vi "GetTrendNames.vi"(11 "AssetNodes":T1[](array[typedef])) -> (3 "trend names":variant)   [LabVIEW 2016]
doc: "Processes the asset nodes for the trend names."
uses:
  <vilib>/addons/InsightCM/Utilities/DeviceModelHelpers/DeviceModelHelpers.lvlib
  <vilib>/addons/InsightCM/MessageBus/Base/controls/AssetState.ctl
  <vilib>/addons/InsightCM/MessageBus/Base/controls/KeyValuePair.ctl
  <vilib>/addons/InsightCM/MessageBus/Base/controls/Metric.ctl
  <vilib>/addons/InsightCM/MessageBus/Base/controls/AssetNodeReference.ctl
  <vilib>/addons/InsightCM/MessageBus/Base/controls/AssetNodeView.ctl
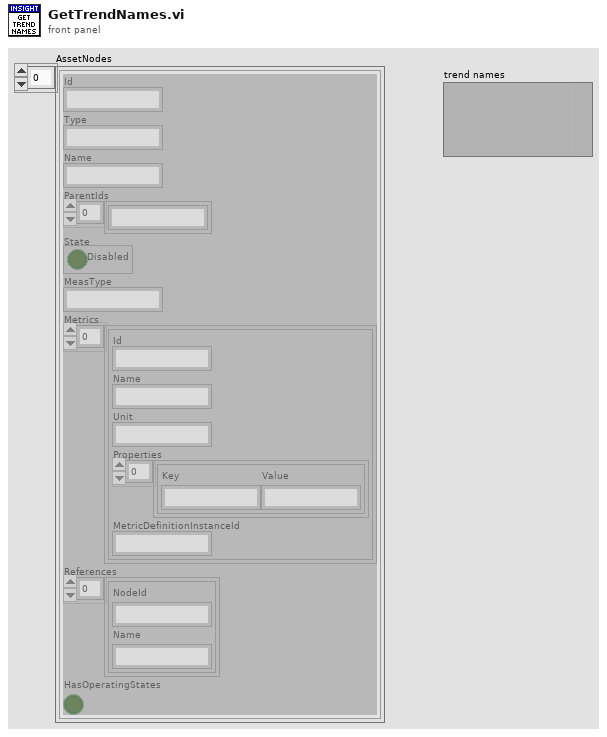
[diagram p1: front panel]
types:
  T1 = typedef "AssetNodeView.ctl" = cluster{"Id":string, "Type":string, "Name":string, "ParentIds":string[], "State":T2, "MeasType":string, "Metrics":T3[], "References":T5[], "HasOperatingStates":bool}
  T2 = typedef "AssetState.ctl" = cluster{"Disabled":bool}
  T3 = typedef "Metric.ctl" = cluster{"Id":string, "Name":string, "Unit":string, "Properties":T4[], "MetricDefinitionInstanceId":string}
  T4 = typedef "KeyValuePair.ctl" = cluster{"Key":string, "Value":string}
  T5 = typedef "AssetNodeReference.ctl" = cluster{"NodeId":string, "Name":string}
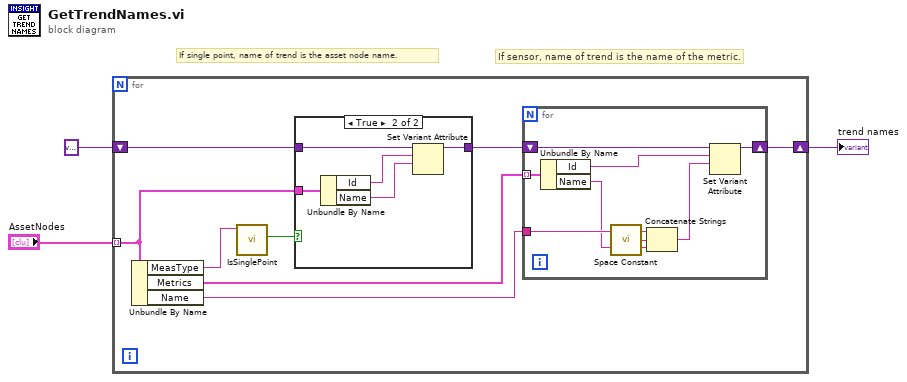
[diagram p0: block diagram]
diagram:
  # "If sensor, name of trend is the name of the metric."
  # "If single point, name of trend is the asset node name."
  n1 = for {
    tunnel: "AssetNodes" -> [w8] mode=indexing
    shift-right: [w6] -> w1
    shift-left: variant ("trend names") -> [w9]
    n2 = Unbundle By Name(w8) -> ("MeasType"=w11:string, "Metrics"=w5:T3[], "Name"=w4:string)
    n3 = call <vilib>:"IsSinglePoint.vi"("MeasType"=w11) -> ("is single point"=w10:bool)  [unwired: 10 in]
    n4 = case shown="True" w10 {
      tunnel: w9 -> [w12 w17]
      tunnel: w8 -> [_ w16]
      tunnel: [w12 w13] -> w7
      frame False {
      }
      frame True {
        n5 = Unbundle By Name(w16) -> ("Id"=w14:string, "Name"=w15:string)
        n6 = Set Variant Attribute(Variant=w17, name=w14, value=w15) -> (Variant out=w13:variant)  [unwired: 1 in, 2 out]
      }
    }
    n7 = for {
      shift-right: [w24] -> w6
      shift-left: w7 -> [w25]
      tunnel: w5 -> [w23] mode=indexing
      tunnel: w4 -> [w20]
      n8 = Unbundle By Name(w23) -> ("Id"=w22:string, "Name"=w19:string)
      n9 = call <vilib>:"Space Constant.vi"() -> ("String"=w21:string)
      n10 = Concatenate Strings(w20, w21, w19) -> (w18:string)
      n11 = Set Variant Attribute(Variant=w25, name=w22, value=w18) -> (Variant out=w24:variant)  [unwired: 1 in, 2 out]
    }
  }
  "trend names" <- w1
